vi "PrepareToPositionBallPlacementSkill.vi"(8 "error in (no error)":errorcluster, 9 "Game":refnum<class "Game.lvclass">, 10 "Robot":refnum<class "Robot.lvclass">, 11 "PrepareToPositionBallPlacementSkill in":refnum<class "PrepareToPositionBallPlacementSkill.lvclass">) -> (0 "error out":errorcluster, 1 "robotCanDoNextAction":bool, 2 "Robot out":refnum<class "Robot.lvclass">, 3 "PrepareToPositionBallPlacementSkill out":refnum<class "PrepareToPositionBallPlacementSkill.lvclass">)   [LabVIEW 2021, in "PrepareToPositionBallPlacementSkill.lvclass"]
uses:
  PrepareToPositionBallPlacementSkill.lvclass
  Robot_class/Robot.lvclass
  D:/RoboIme/horie/SSL_AI/Object_class/Object.lvclass
  Game_class/Game.lvclass
  Object_class/Object.lvclass/Object.ctl
  Game_class/Game.lvclass/Game.ctl
  Robot_class/Robot.lvclass/Robot.ctl
  Game_class/Read FieldRef.vi
  Game_class/Read Referee.vi
  Game_class/Read BallRef.vi
  Game_class/Read Parameters.lvclass.vi
  Object_class/Read position(x,y).vi
  Robot_class/Write dest_x.vi
  Robot_class/Write dest_y.vi
  Robot_class/Write dest_orientation.vi
  Robot_class/Write dribble.vi
  Field_class/Field.lvclass
  Referee_class/Referee.lvclass
  Ball_class/Ball.lvclass
  Parameters_class/Parameters.lvclass
  Utilities_class/Utilities.lvclass
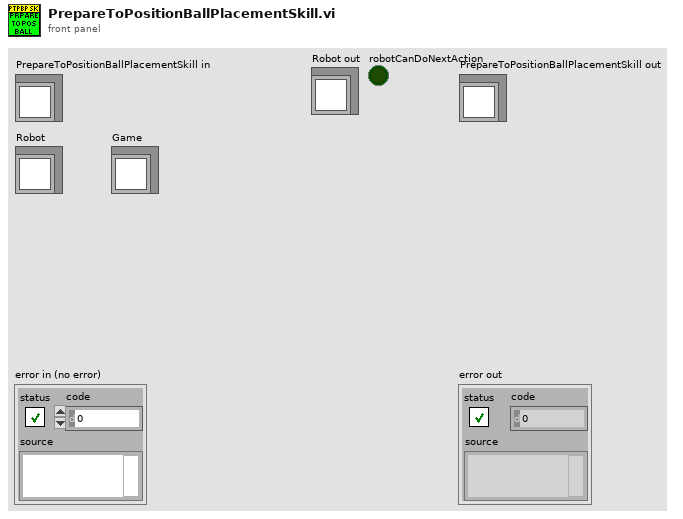
[diagram p1: front panel]
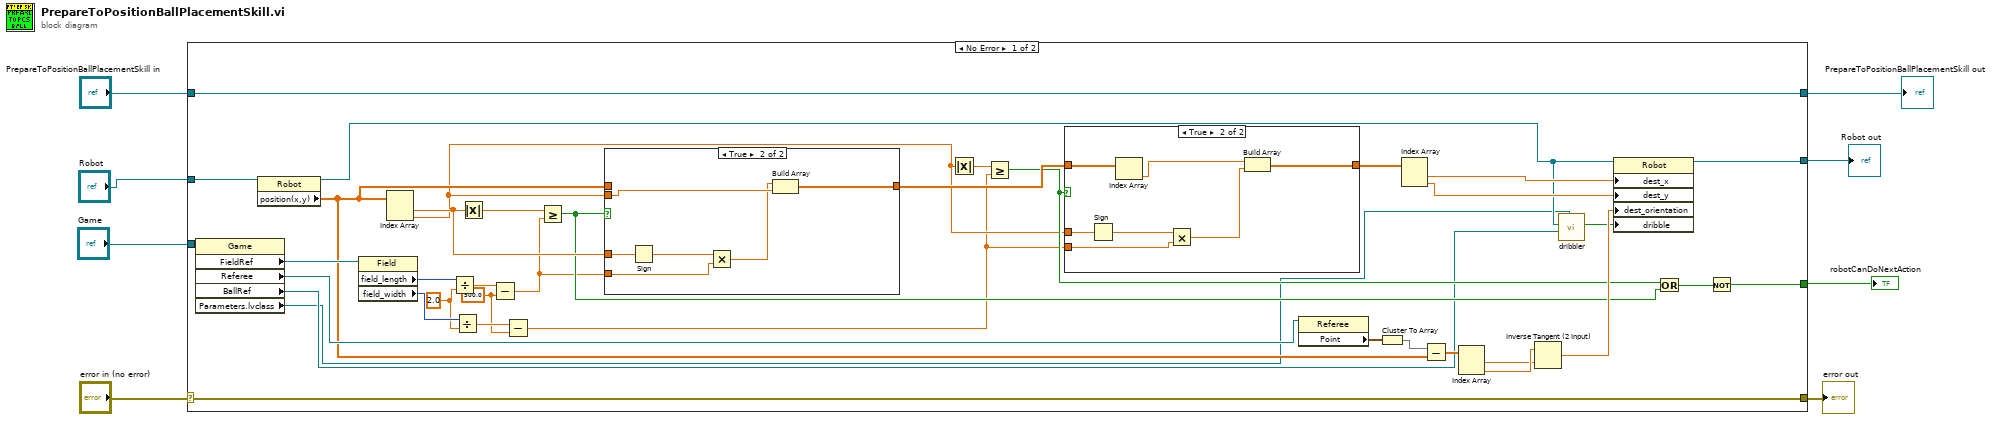
[diagram p0: block diagram]
diagram:
  n1 = case shown="No Error" "error in (no error)" {
    selector: "error in (no error)" -> [w46 w63]
    tunnel: [w46 w63] -> w7
    tunnel: [w38 w62] -> w5
    tunnel: "PrepareToPositionBallPlacementSkill in" -> [w38 w62]
    tunnel: "Robot" -> [w45 _]
    tunnel: "Game" -> [w43 _]
    tunnel: [w28 _] -> w2
    tunnel: [w16 _] -> w1
    frame No Error {
      w32 = 500.0 ("y")
      w35 = 2.0
      n2 = property class="Game"(reference=w43) -> ("FieldRef"=w42:refnum<class "Field.lvclass">, "Referee"=w27:refnum<class "Referee.lvclass">, "BallRef"=w10:refnum<class "Ball.lvclass">, "Parameters.lvclass"=w9:refnum<class "Parameters.lvclass">)  [unwired: 1 in, 2 out]
      n3 = property class="Robot"(reference=w45) -> (reference out=w11:refnum<class "Robot.lvclass">, "position(x,y)"=w25:dbl[])  [unwired: 1 in, 1 out]
      n4 = property class="Field"(reference=w42) -> ("field_length"=w41:i32, "field_width"=w36:i32)  [unwired: 1 in, 2 out]
      n5 = Index Array(array=w25) -> (element #1=w39:dbl, element #2=w15:dbl)  [unwired: 2 in]
      n6 = Divide(x=w41, y=w35) -> (x/y=w40:dbl)
      n7 = Divide(x=w36, y=w35) -> (x/y=w34:dbl)
      n8 = Absolute Value(x=w39) -> (abs(x)=w44:dbl)
      n9 = Subtract(x=w40, y=w32) -> (x-y=w14:dbl)
      n10 = Subtract(x=w34, y=w32) -> (x-y=w13:dbl)
      n11 = Greater Or Equal?(x=w44, y=w14) -> (x >= y?=w19:bool)
      n12 = case shown="True" w19 {
        tunnel: w25 -> [w55 _]
        tunnel: w39 -> [_ w61]
        tunnel: [w55 w60] -> w33
        tunnel: w15 -> [_ w59]
        tunnel: w14 -> [_ w58]
        frame False {
        }
        frame True {
          n13 = Sign(1:w61) -> (0:w56:dbl)
          n14 = Multiply(x=w56, y=w58) -> (x*y=w57:dbl)
          n15 = Build Array(w57, w59) -> (w60:dbl[])
        }
      }
      n16 = Absolute Value(x=w15) -> (abs(x)=w37:dbl)
      n17 = Greater Or Equal?(x=w37, y=w13) -> (x >= y?=w18:bool)
      n18 = case shown="True" w18 {
        tunnel: w33 -> [w47 w52]
        tunnel: w15 -> [_ w54]
        tunnel: [w47 w50] -> w31
        tunnel: w13 -> [_ w48]
        frame False {
        }
        frame True {
          n19 = Sign(1:w54) -> (0:w53:dbl)
          n20 = Index Array(array=w52) -> (element=w51:dbl)  [unwired: 1 in]
          n21 = Multiply(x=w53, y=w48) -> (x*y=w49:dbl)
          n22 = Build Array(w51, w49) -> (w50:dbl[])
        }
      }
      n23 = property class="Referee"(reference=w27) -> ("Point"=w26:cluster{"x":sgl, "y":sgl})  [unwired: 1 in, 2 out]
      n24 = Cluster To Array(cluster=w26) -> (array=w24:sgl[])
      n25 = Index Array(array=w31) -> (element #1=w30:dbl, element #2=w29:dbl)  [unwired: 2 in]
      n26 = Subtract(x=w24, y=w25) -> (x-y=w23:dbl[])
      n27 = Index Array(array=w23) -> (element #1=w21:dbl, element #2=w22:dbl)  [unwired: 2 in]
      n28 = Inverse Tangent (2 Input)(1:w21, 2:w22) -> (0:w20:dbl)
      n29 = call "dribbler.vi"("Parameters.lvclass"=w9, "Ball"=w10, "Robot"=w11) -> ("Dribbler?"=w12:bool)  [unwired: 6 in, 2 out]
      n30 = property class="Robot"(reference=w11, "dest_x"=w30, "dest_y"=w29, "dest_orientation"=w20, "dribble"=w12) -> (reference out=w28:refnum<class "Robot.lvclass">)  [unwired: 1 in, 1 out]
      n31 = Or(x=w18, y=w19) -> (x .or. y?=w17:bool)
      n32 = Not(x=w17) -> (.not. x?=w16:bool)
    }
    frame Error {
    }
  }
  "error out" <- w7
  "PrepareToPositionBallPlacementSkill out" <- w5
  "Robot out" <- w2
  "robotCanDoNextAction" <- w1
